vi "Telnet_Close.vi"(8 "Error In":errorcluster caption="Entrée d'erreur", 11 "telnet connection":T1) -> (0 "Error Out":errorcluster caption="Sortie d'erreur", 3 "Connecté":bool)   [LabVIEW 2013]
uses:
  <vilib>/addons/internet/telnet/telnet.llb/Telnet Session.ctl
  <vilib>/addons/internet/NI_InternetTK_Core_VIs.lvlib
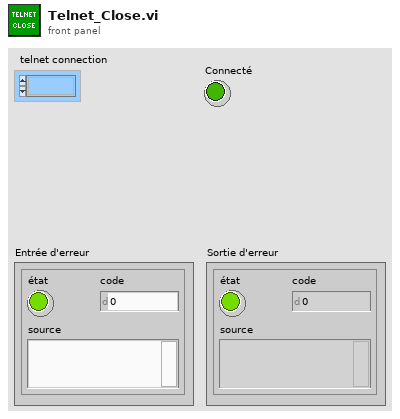
[diagram p1: front panel]
types:
  T1 = typedef "Telnet Session.ctl" = refnum<k1>
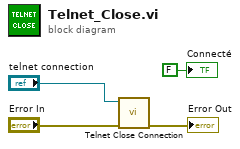
[diagram p0: block diagram]
diagram:
  n1 = call <vilib>:"Telnet Close Connection.vi"("error in (no error)"="Error In", "telnet connection"="telnet connection") -> ("error out"=→"Error Out":errorcluster)  [unwired: 8 in, 1 out]
  "Connecté" <- FALSE ("Déconnecté")
